vi "Line Detector Initial Guess from Peak Findervi.vi"(6 "Peak finder guess":dbl[](array[numeric]), 10 "Signal":cdb[](array[numeric])) -> (3 "Initial guess":dbl[](array[numeric]))   [LabVIEW 2016]
panel:
  # "F0         dF     Ampl   Phase   Xbgrd   Ybgrd       mask"
  # "F0\n\nWidth\n\nAmpl"
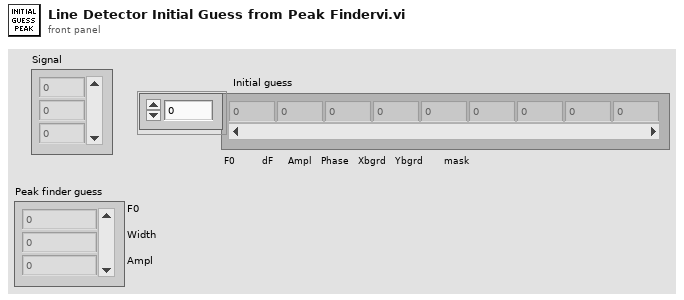
[diagram p1: front panel]
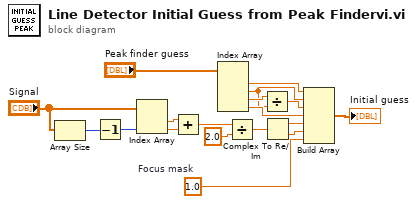
[diagram p0: block diagram]
diagram:
  w1 = 1.0  # Focus mask
  n1 = Array Size(array="Signal") -> (size(s)=w17:i32)
  n2 = Decrement(x=w17) -> (x-1=w16:i32)
  n3 = Index Array(array="Signal", index #2=w16) -> (element #1=w15:cdb, element #2=w14:cdb)  [unwired: 1 in]
  n4 = Add(x=w15, y=w14) -> (x+y=w13:cdb)
  n5 = Index Array(array="Peak finder guess") -> (element #1=w10:dbl, element #2=w3:dbl, element #3=w4:dbl, element #4=w6:dbl)  [unwired: 4 in]
  n6 = Divide(x=w13, y=2.0) -> (x/y=w9:cdb)
  n7 = Divide(x=w4, y=w3) -> (x/y=w2:dbl)
  n8 = Complex To Re/Im(x + iy=w9) -> (x=w12:dbl, y=w11:dbl)
  n9 = Build Array(w10, w3, w2, w6, w12, w11, w1) -> (→"Initial guess":dbl[])
